vi "Get User Interface VI.vi"(8 "error in (no error)":errorcluster, 11 "UDP Thread User Interface in":refnum<class "UDP Thread User Interface.lvclass">) -> (0 "error out":errorcluster, 2 "user interface vi":refnum<vi>, 3 "UDP Thread User Interface out":refnum<class "UDP Thread User Interface.lvclass">)   [LabVIEW 2017, in "UDP Transceiver.lvlib" / "UDP Thread User Interface.lvclass"]
uses:
  UDP Thread User Interface.lvclass
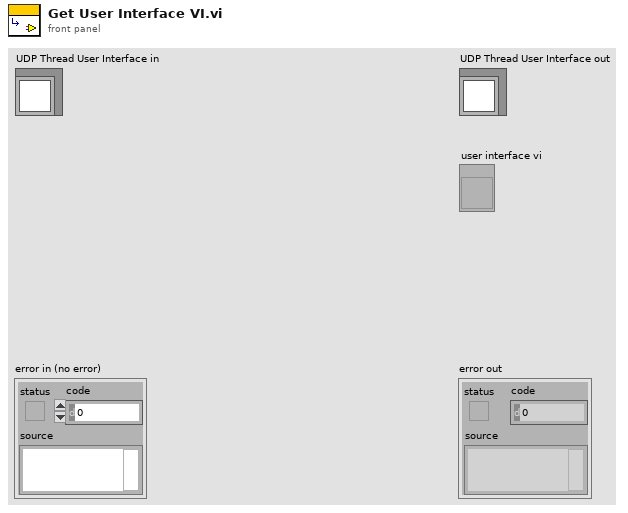
[diagram p1: front panel]
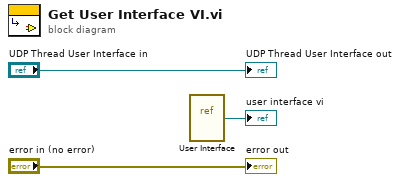
[diagram p0: block diagram]
diagram:
  n1 = vi-ref "User Interface.vi"() -> (→"user interface vi":refnum<vi>)
  "error out" <- "error in (no error)"
  "UDP Thread User Interface out" <- "UDP Thread User Interface in"
